vi "Load Mov Dev config.vi"(7 "Montura":T2, 8 "error in (no error)":errorcluster, 10 "Datos Adquisición":T1={"Equipo a Utilizar"=enum."TDS 2012B Osciloscope", "Montura"=enum."Zaber T-LSR450B", "Datos Zaber"={"Sentido de Adquisición"=TRUE, "Comenzar Desde Home?"=TRUE, "Distancia a recorrer (um)"=10.0, "Pasos motor"=0, "Distancia entre Lecturas (um)"=0.1, "Puerto"="UNKNOWN"}, "Datos Bipolar/Unipolar"={"Puerto COM"="UNKNOWN", "Pasos entre Lecturas"=0, "Numero de lecturas"=0, "Sentido del motor"=TRUE}, "Datos Archivo"={"Ruta Archivo"=path "", "Nombre de Prueba"=""}, "Datos actuales"={"Montura"="", "Equipo"="", "Posición Actual"="", "Distancia Total a recorrer"="", "distancia Entre lecturas"="", "Pasos entre lecturas"=""}, "Datos a Guardar In"={"Datos Cursor Tektronix"="", "Datos Lokin"="", "Posición Cero"=0.0, "Posición Actual"=0.0}, "Datos Osciloscopio"={"Sesión Visa Osciloscopio"="UNKNOWN", "Tipo de Adquisición"=enum."Voltaje Pico Pico", "Canal a Utilizar"=enum."Canal 1", "Parametros de Adquisición"=enum."Una Muestra", "Número Promedio"=2}, "Datos Lock In"={"Visa Lock in"="Tektronix_TDS2012C"}} {"Datos Osciloscopio"."Número Promedio" min=2 max=20; "Datos a Guardar In"."Posición Actual" format="%#_10f"; "Datos a Guardar In"."Posición Cero" format="%#_10f"; "Datos Bipolar/Unipolar"."Numero de lecturas" max=910098 step=1}, 11 "Refnum in":T7) -> (0 "error out":errorcluster, 1 "Valid?":bool, 2 "Datos Adquisición out":T1={"Equipo a Utilizar"=enum."TDS 2012B Osciloscope", "Montura"=enum."Zaber T-LSR450B", "Datos Zaber"={"Sentido de Adquisición"=TRUE, "Comenzar Desde Home?"=TRUE, "Distancia a recorrer (um)"=10.0, "Pasos motor"=0, "Distancia entre Lecturas (um)"=0.1, "Puerto"="UNKNOWN"}, "Datos Bipolar/Unipolar"={"Puerto COM"="UNKNOWN", "Pasos entre Lecturas"=0, "Numero de lecturas"=0, "Sentido del motor"=TRUE}, "Datos Archivo"={"Ruta Archivo"=path "", "Nombre de Prueba"=""}, "Datos actuales"={"Montura"="", "Equipo"="", "Posición Actual"="", "Distancia Total a recorrer"="", "distancia Entre lecturas"="", "Pasos entre lecturas"=""}, "Datos a Guardar In"={"Datos Cursor Tektronix"="", "Datos Lokin"="", "Posición Cero"=0.0, "Posición Actual"=0.0}, "Datos Osciloscopio"={"Sesión Visa Osciloscopio"="UNKNOWN", "Tipo de Adquisición"=enum."Voltaje Pico Pico", "Canal a Utilizar"=enum."Canal 1", "Parametros de Adquisición"=enum."Una Muestra", "Número Promedio"=2}, "Datos Lock In"={"Visa Lock in"="Tektronix_TDS2012C"}} {"Datos Osciloscopio"."Número Promedio" min=2 max=20; "Datos a Guardar In"."Posición Actual" format="%#_10f"; "Datos a Guardar In"."Posición Cero" format="%#_10f"; "Datos Bipolar/Unipolar"."Numero de lecturas" max=910098 step=1}, 3 "refnum out":T7)   [LabVIEW 2020]
uses:
  Type Definitions/parametros motores.ctl
  Type Definitions/Datos Zaber.ctl
  <vilib>/Utility/config.llb/NI_LVConfig.lvlib
  <vilib>/Utility/config.llb/Read Key (String).vi
  <vilib>/Utility/config.llb/Read Key (Double).vi
  <vilib>/Utility/config.llb/Read Key (Boolean).vi
  <vilib>/Utility/config.llb/Read Key (U32).vi
  <vilib>/Utility/config.llb/Config Data RefNum.ctl
  H:/Mi unidad/Departamento de Ingenieria/Investigadores/Gabriel Ramos/Proyecto Monturas v13/LV Source/Type Definitions/Tipos de montura.ctl
  Type Definitions/Datos a Guardar.ctl
  Type Definitions/datos osciloscopio.ctl
  Type Definitions/Asistente de adquisicion Cluster.ctl
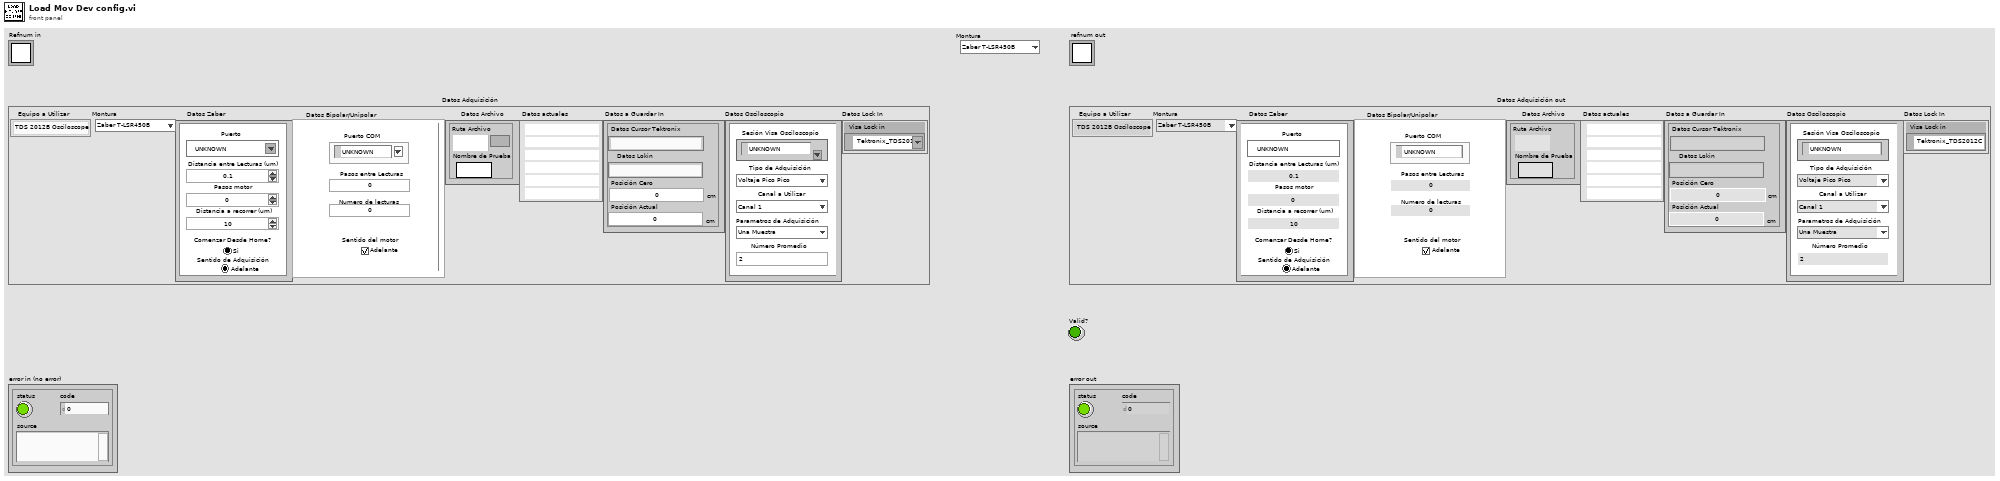
[diagram p1: front panel]
types:
  T1 = typedef "Asistente de adquisicion Cluster.ctl" = cluster{"Equipo a Utilizar":enum16{"SR830 Lock In", "TDS 2012B Osciloscope"}, "Montura":T2, "Datos Zaber":T3, "Datos Bipolar/Unipolar":T4, "Datos Archivo":cluster{"Ruta Archivo":path, "Nombre de Prueba":string}, "Datos actuales":cluster{"Montura":string, "Equipo":string, "Posición Actual":string, "Distancia Total a recorrer":string, "distancia Entre lecturas":string, "Pasos entre lecturas":string}, "Datos a Guardar In":T5, "Datos Osciloscopio":T6, "Datos Lock In":cluster{"Visa Lock in":refnum<visa-resource-name>}}
  T2 = typedef "Tipos de montura.ctl" = enum16{"Zaber T-LSR450B", "Zaber-T-LSR300B", "Zaber-T-LSRxxx", "Motor Bipolar", "Motor Unipolar"}
  T3 = typedef "Datos Zaber.ctl" = cluster{"Sentido de Adquisición":bool, "Comenzar Desde Home?":bool, "Distancia a recorrer (um)":dbl, "Pasos motor":i32, "Distancia entre Lecturas (um)":dbl, "Puerto":refnum<visa-resource-name>}
  T4 = typedef "parametros motores.ctl" = cluster{"Puerto COM":refnum<visa-resource-name>, "Pasos entre Lecturas":u16, "Numero de lecturas":u32, "Sentido del motor":bool}
  T5 = typedef "Datos a Guardar.ctl" = cluster{"Datos Cursor Tektronix":string, "Datos Lokin":string, "Posición Cero":dbl[unit], "Posición Actual":dbl[unit]}
  T6 = typedef "datos osciloscopio.ctl" = cluster{"Sesión Visa Osciloscopio":refnum<visa-resource-name>, "Tipo de Adquisición":enum16{"Voltaje Pico Pico", "Voltaje RMS", "Cursor Tiempo"}, "Canal a Utilizar":enum16{"Canal 1", "Canal 2", "Canal 1 y 2"}, "Parametros de Adquisición":enum16{"Una Muestra", "Promedio"}, "Número Promedio":i32}
  T7 = typedef "NI_LVConfig.lvlib/Config Data RefNum.ctl" = refnum<k1>
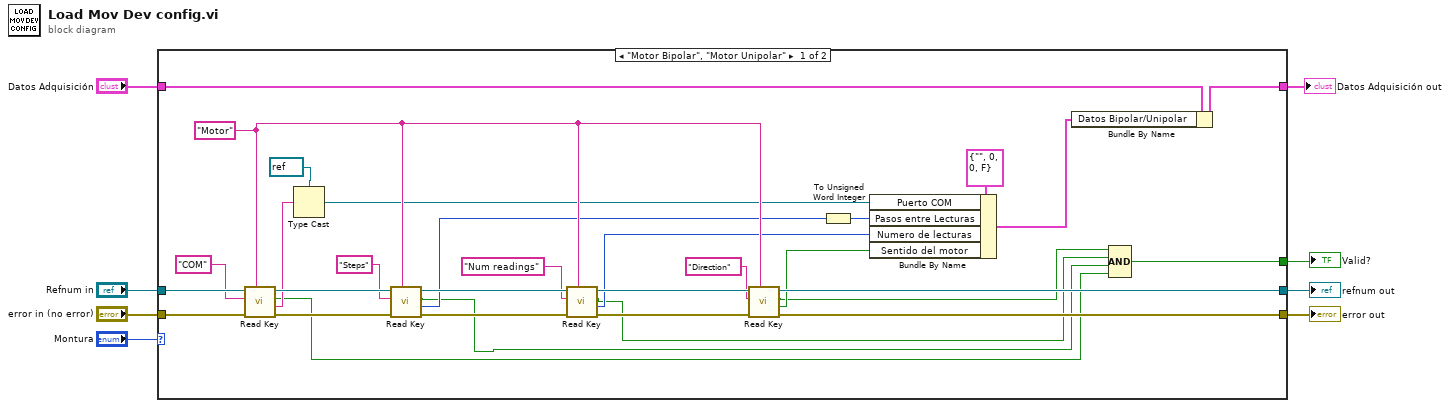
[diagram p0: block diagram]
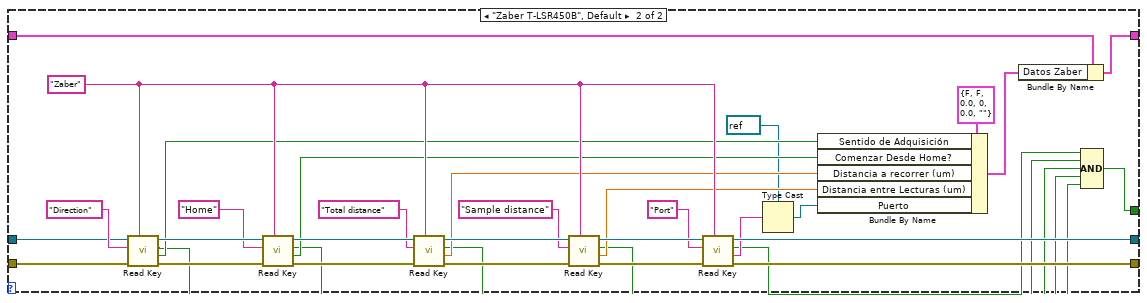
[diagram p2: hidden frame]
diagram:
  n1 = case shown="\"Motor Bipolar\", \"Motor Unipolar\"" "Montura" {
    tunnel: "Refnum in" -> [w38 w71]
    tunnel: "error in (no error)" -> [w39 w74]
    tunnel: [w29 w61] -> w5
    tunnel: [w27 w59] -> w4
    tunnel: "Datos Adquisición" -> [w16 w48]
    tunnel: [w14 w46] -> w2
    tunnel: [w9 w40] -> w1
    frame "Motor Bipolar", "Motor Unipolar" {
      w26 = "Motor" ("section")
      n2 = call-poly <vilib>:"Read Key.vi"("section"=w26, "error in (no error)"=w39, "key"="COM", "refnum"=w38) -> ("error out"=w37:errorcluster, "value"=w23:string, "found?"=w13:bool, "refnum out"=w35:T7)  [unwired: 4 in]
      n3 = Type Cast(type=refnum<visa-resource-name> refnum ("Puerto COM"), x=w23) -> (*(type *) &x=w21:refnum<visa-resource-name>)
      n4 = call-poly <vilib>:"Read Key.vi"("section"=w26, "error in (no error)"=w37, "key"="Steps", "refnum"=w35) -> ("error out"=w36:errorcluster, "value"=w20:u32, "found?"=w12:bool, "refnum out"=w32:T7)  [unwired: 4 in]
      n5 = call-poly <vilib>:"Read Key.vi"("section"=w26, "error in (no error)"=w36, "key"="Num readings", "refnum"=w32) -> ("error out"=w30:errorcluster, "value"=w18:u32, "found?"=w11:bool, "refnum out"=w28:T7)  [unwired: 4 in]
      n6 = call-poly <vilib>:"Read Key.vi"("section"=w26, "error in (no error)"=w30, "key"="Direction", "refnum"=w28) -> ("error out"=w29:errorcluster, "value"=w17:bool, "found?"=w10:bool, "refnum out"=w27:T7)  [unwired: 4 in]
      n7 = To Unsigned Word Integer(number=w20) -> (unsigned 16bit integer=w19:u16)
      n8 = Bundle By Name(cluster=T4 {"Puerto COM"="", "Pasos entre Lecturas"=0, "Numero de lecturas"=0, "Sentido del motor"=FALSE} ("Datos Bipolar/Unipolar"), "Puerto COM"=w21, "Pasos entre Lecturas"=w19, "Numero de lecturas"=w18, "Sentido del motor"=w17) -> (w15:T4)
      n9 = Bundle By Name(cluster=w16, "Datos Bipolar/Unipolar"=w15) -> (w14:T1)
      n10 = Compound Arithmetic op=AND(w10, w11, w12, w13) -> (w9:bool)
    }
    frame "Zaber T-LSR450B", Default {
      w58 = "Zaber" ("section")
      n11 = call-poly <vilib>:"Read Key.vi"("section"=w58, "error in (no error)"=w74, "key"="Direction", "refnum"=w71) -> ("error out"=w73:errorcluster, "value"=w55:bool, "found?"=w45:bool, "refnum out"=w69:T7)  [unwired: 4 in]
      n12 = call-poly <vilib>:"Read Key.vi"("section"=w58, "error in (no error)"=w73, "key"="Home", "refnum"=w69) -> ("error out"=w70:errorcluster, "value"=w54:bool, "found?"=w44:bool, "refnum out"=w66:T7)  [unwired: 4 in]
      n13 = call-poly <vilib>:"Read Key.vi"("section"=w58, "error in (no error)"=w70, "key"="Total distance", "refnum"=w66) -> ("error out"=w67:errorcluster, "value"=w53:dbl, "found?"=w43:bool, "refnum out"=w63:T7)  [unwired: 4 in]
      n14 = call-poly <vilib>:"Read Key.vi"("section"=w58, "error in (no error)"=w67, "key"="Sample distance", "refnum"=w63) -> ("error out"=w64:errorcluster, "value"=w52:dbl, "found?"=w42:bool, "refnum out"=w60:T7)  [unwired: 4 in]
      n15 = call-poly <vilib>:"Read Key.vi"("section"=w58, "error in (no error)"=w64, "key"="Port", "refnum"=w60) -> ("error out"=w61:errorcluster, "value"=w51:string, "found?"=w41:bool, "refnum out"=w59:T7)  [unwired: 4 in]
      n16 = Type Cast(type=refnum<visa-resource-name> refnum ("Puerto"), x=w51) -> (*(type *) &x=w49:refnum<visa-resource-name>)
      n17 = Bundle By Name(cluster=T3 {"Sentido de Adquisición"=FALSE, "Comenzar Desde Home?"=FALSE, "Distancia a recorrer (um)"=0.0, "Pasos motor"=0, "Distancia entre Lecturas (um)"=0.0, "Puerto"=""} ("Datos Zaber"), "Sentido de Adquisición"=w55, "Comenzar Desde Home?"=w54, "Distancia a recorrer (um)"=w53, "Distancia entre Lecturas (um)"=w52, "Puerto"=w49) -> (w47:T3)
      n18 = Bundle By Name(cluster=w48, "Datos Zaber"=w47) -> (w46:T1)
      n19 = Compound Arithmetic op=AND(w41, w42, w43, w44, w45) -> (w40:bool)
    }
  }
  "error out" <- w5
  "refnum out" <- w4
  "Datos Adquisición out" <- w2
  "Valid?" <- w1
